vi "InsideTile.vi"(4 "index_y":u16, 6 "index_x":u16, 7 "TileNo":u8, 9 "Rotate":u8, 10 "pos_y":u16, 11 "pos_x":u16) -> (2 "TilePixelIndex":u16, 3 "InsideTile?":bool)   [LabVIEW 2019, in "Tiles.lvlib"]
doc: "Decides if index_x and index_y are in range of the tile. Calculates the coordinate of the Tile based on rotation."
uses:
  Tiles.lvlib
  ded9a89c-2383-4f36-919f-3b6d0360cd66.vi
  5b7b7b12-061c-4b47-b5d5-7aa3a6fff0a0.vi
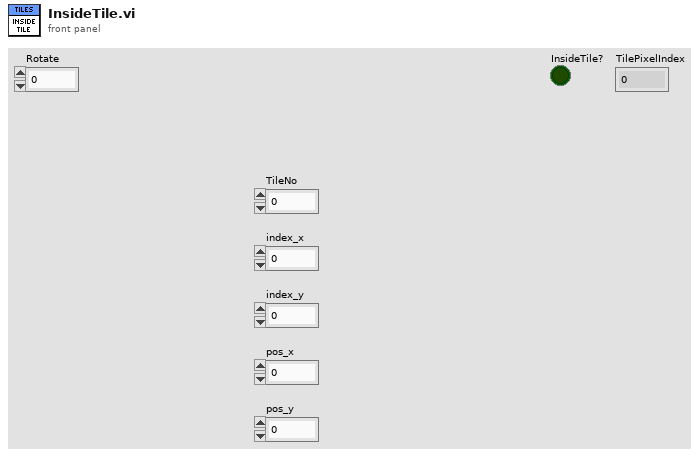
[diagram p1: front panel]
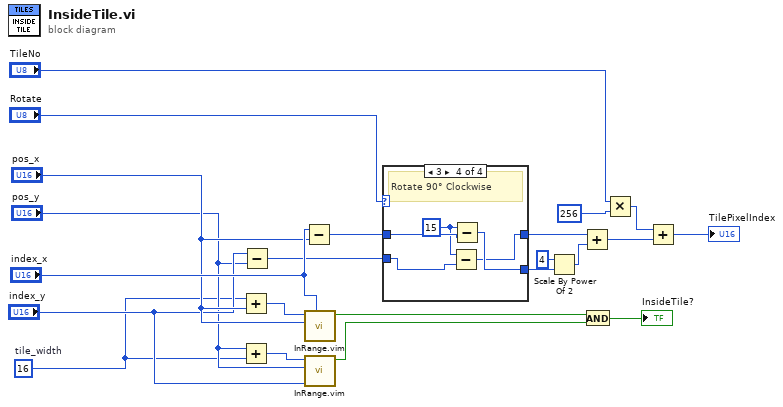
[diagram p0: block diagram]
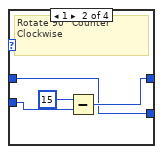
[diagram p3: hidden frame]
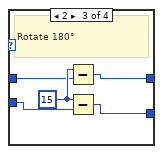
[diagram p4: hidden frame]
diagram:
  w9 = u16 16  # tile_width
  n1 = Add(x=w9, y="pos_x") -> (x+y=w20:u16)
  n2 = Add(x="pos_y", y=w9) -> (x+y=w19:u16)
  n3 = Subtract(x="index_y", y="pos_y") -> (x-y=w2:u16)
  n4 = Subtract(x="index_x", y="pos_x") -> (x-y=w5:u16)
  n5 = call "InRange.vim"("x"="index_x", "Low"="pos_x", "Up"=w20) -> ("InRange?"=w15:bool)  [unwired: 8 in]
  n6 = call "InRange.vim"("x"="index_y", "Low"="pos_y", "Up"=w19) -> ("InRange?"=w14:bool)  [unwired: 8 in]
  n7 = case shown="3" "Rotate" {
    tunnel: w5 -> [w24 w25 w31 w38]
    tunnel: [w24 w26 w30 w35] -> w4
    tunnel: [w23 w25 w29 w37] -> w3
    tunnel: w2 -> [w23 w28 w33 w36]
    frame 0, Default {
    }
    frame 1 {
      # "Rotate 90° Counter Clockwise"
      n8 = Subtract(x=u16 15, y=w28) -> (x-y=w26:u16)
    }
    frame 2 {
      w32 = u16 15 ("x")
      # "Rotate 180°"
      n9 = Subtract(x=w32, y=w31) -> (x-y=w30:u16)
      n10 = Subtract(x=w32, y=w33) -> (x-y=w29:u16)
    }
    frame 3 {
      w34 = u16 15 ("x")
      # "Rotate 90° Clockwise"
      n11 = Subtract(x=w34, y=w36) -> (x-y=w35:u16)
      n12 = Subtract(x=w34, y=w38) -> (x-y=w37:u16)
    }
  }
  n13 = Scale By Power Of 2(n=i16 4, x=w3) -> (x*2^n=w22:u16)
  n14 = Add(x=w4, y=w22) -> (x+y=w21:u16)
  n15 = And(x=w15, y=w14) -> (x .and. y?=→"InsideTile?":bool)
  n16 = Multiply(x="TileNo", y=u16 256) -> (x*y=w16:u16)
  n17 = Add(x=w16, y=w21) -> (x+y=→"TilePixelIndex":u16)
